vi "rohitRS.vi"() -> ()   [LabVIEW 2009]
panel:
  out "A3":dbl
  in  "Serial Data Input":dbl
  out "A0":dbl
  out "A1":dbl
  out "A2":dbl
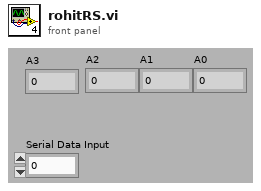
[diagram p1: front panel]
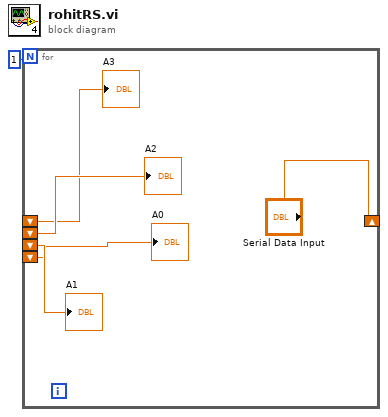
[diagram p0: block diagram]
diagram:
  n1 = for {
    N: 1 -> [_]
    shift-right: ["Serial Data Input"] -> _
    shift-left: _ -> [w3]
    shift-left: _ -> [w6]
    shift-left: _ -> [w5]
    shift-left: _ -> [w4]
    "A2" <- w6
    "A1" <- w5
    "A0" <- w4
    "A3" <- w3
  }
